vi "Read Command Response.vi"(8 "error in (no error)":errorcluster, 10 "Shell Command":string, 11 "Resource in":refnum<class "DeployResource.lvclass">) -> (0 "error out":errorcluster, 2 "Value":string, 3 "Resource out":refnum<class "DeployResource.lvclass">)   [LabVIEW 2020, in "PicoG-Core.lvlib" / "DeployResource.lvclass"]
uses:
  DeployResource.lvclass
  PicoG-Core.lvlib
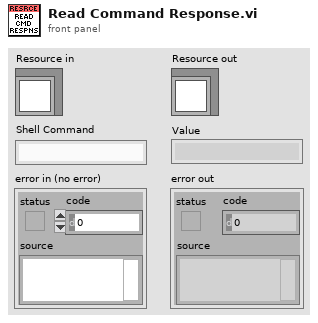
[diagram p1: front panel]
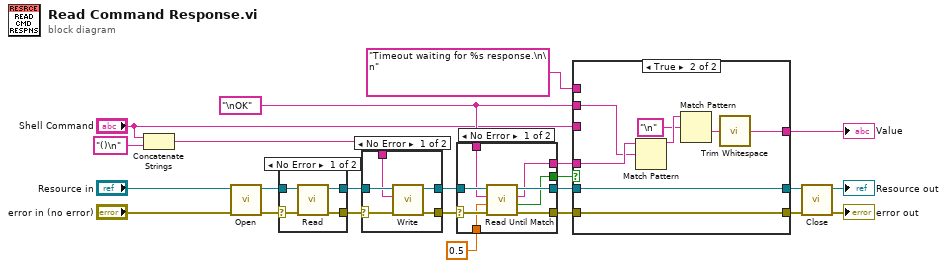
[diagram p0: block diagram]
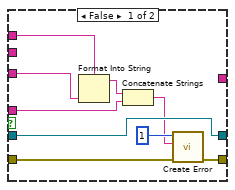
[diagram p3: hidden frame]
diagram:
  w16 = "\nOK" ("Data")
  n1 = Concatenate Strings("Shell Command", "()\n" ("Data")) -> (w2:string)
  n2 = call-dynamic "Open.vi"("error in (no error)"="error in (no error)", "DeployResource in"="Resource in") -> ("error out"=w12:errorcluster, "DeployResource out"=w11:refnum<class "DeployResource.lvclass">)  [unwired: 8 in]
  n3 = case shown="No Error" w12 {
    selector: w12 -> [w27 w29]
    tunnel: w11 -> [w26 w28]
    tunnel: [w25 w29] -> w10
    tunnel: [w24 w28] -> w9
    frame No Error {
      n4 = call "Read.vi"("error in (no error)"=w27, "DeployResource in"=w26) -> ("error out"=w25:errorcluster, "DeployResource out"=w24:refnum<class "DeployResource.lvclass">)  [unwired: 6 in, 2 out]
    }
    frame Error {
    }
  }
  n5 = case shown="No Error" w10 {
    selector: w10 -> [w33 w35]
    tunnel: w9 -> [w34 w36]
    tunnel: w2 -> [w32 _]
    tunnel: [w31 w36] -> w23
    tunnel: [w30 w35] -> w22
    frame No Error {
      n6 = call "Write.vi"("error in (no error)"=w33, "Data"=w32, "DeployResource in"=w34) -> ("error out"=w30:errorcluster, "DeployResource out"=w31:refnum<class "DeployResource.lvclass">)  [unwired: 6 in, 1 out]
    }
    frame Error {
    }
  }
  n7 = case shown="No Error" w22 {
    selector: w22 -> [w43 w46]
    tunnel: w23 -> [w44 w45]
    tunnel: 0.5 ("Timeout S (0)") -> [w42 _]
    tunnel: [w40 w46] -> w20
    tunnel: [w41 w45] -> w19
    tunnel: w16 -> [w39 _]
    tunnel: [w38 _] -> w18
    tunnel: [w37 _] -> w17
    frame No Error {
      n8 = call "Read Until Match.vi"("error in (no error)"=w43, "Timeout S (0)"=w42, "Match String"=w39, "DeployResource in"=w44) -> ("error out"=w40:errorcluster, "Found?"=w38:bool, "Data"=w37:string, "DeployResource out"=w41:refnum<class "DeployResource.lvclass">)  [unwired: 4 in]
    }
    frame Error {
    }
  }
  n9 = case shown="True" w18 {
    tunnel: w19 -> [w53 w59]
    tunnel: w20 -> [w55 w58]
    tunnel: w17 -> [w51 w63]
    tunnel: w16 -> [_ w62]
    tunnel: [_ w56] -> w4
    tunnel: [w53 w59] -> w13
    tunnel: [w54 w58] -> w14
    tunnel: "Timeout waiting for %s response.\n\n" ("Message (\"\")") -> [w49 _]
    tunnel: "Shell Command" -> [w48 _]
    frame False {
      n10 = Format Into String(format string=w49, w48) -> (resulting string=w47:string)  [unwired: 2 in, 1 out]
      n11 = Concatenate Strings(w47, w51) -> (w50:string)
      n12 = call "Create Error.vi"("error in (no error)"=w55, "Message (\"\")"=w50, "Code"=1) -> ("error out"=w54:errorcluster)  [unwired: 8 in]
    }
    frame True {
      n13 = Match Pattern(string=w63, regular expression=w62) -> (before substring=w61:string)  [unwired: 1 in, 3 out]
      n14 = Match Pattern(string=w61, regular expression="\n" ("Data")) -> (after substring=w57:string)  [unwired: 1 in, 3 out]
      n15 = call <vilib>:"Trim Whitespace.vi"("string"=w57) -> ("trimmed string"=w56:string)  [unwired: 1 in]
    }
  }
  "Value" <- w4
  n16 = call-dynamic "Close.vi"("error in (no error)"=w14, "DeployResource in"=w13) -> ("error out"=→"error out":errorcluster, "DeployResource out"=→"Resource out":refnum<class "DeployResource.lvclass">)  [unwired: 8 in]
